vi "MHX Tube Heat Transfer Coefficient.vi"(6 "MHX Pri Re":dbl, 7 "MHX Pri Pr":dbl, 9 "MHX Pri Phi":dbl, 10 "Pipe Diameter":dbl, 11 "Thermal Conductivity of FLiBe":dbl) -> (3 "MHX Tube h":dbl)   [LabVIEW 2019]
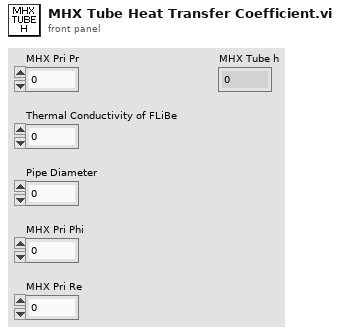
[diagram p1: front panel]
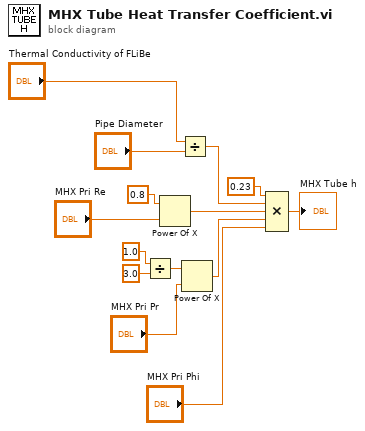
[diagram p0: block diagram]
diagram:
  n1 = Divide(x=1.0, y=3.0) -> (x/y=w10:dbl)
  n2 = Power Of X(1:"MHX Pri Re", 2:0.8 ("y")) -> (0:w7:dbl)
  n3 = Divide(x="Thermal Conductivity of FLiBe", y="Pipe Diameter") -> (x/y=w4:dbl)
  n4 = Power Of X(1:"MHX Pri Pr", 2:w10) -> (0:w12:dbl)
  n5 = Compound Arithmetic op=MULTIPLY(0.23 ("value"), w4, w7, w12, "MHX Pri Phi") -> (→"MHX Tube h":dbl)
